vi "main--material example.vi"() -> ()   [LabVIEW 2021]
doc: "Example UI VI -- shows a couple example buttons and how to use the load and application VIs to theme the sample UI\n\n<b>Code Developed By:</b>\nTechnology Service Corporation\nwww.tsc.com/atcs\n\nDeveloper:\nDaniel Coons"
uses:
  src/Material Theme/Material Theme.lvclass
  user32.dll
panel:
  in  "tab control--Inverse Primary":enum32{"Page 1", "Page 2"}(tab)
  in  "File Path (theme)":path
  in  "theme-switch":bool
  out "status":string
  in  "filled--text--rectangular":bool
  in  "tonal--icons--rounded":bool
  in  "outline--text--rectangular":bool
  in  "FAB Button":bool
  in  "Close":bool
  out "header":bool
  # "control UI role = Secondary"
  # "Note:  run the VI to see dynamic theme in action!"
  # "Front Panel Rule: Surface"
  # "control UI role = Primary"
  # "control UI role = Primary"
  # "Decoration--Surface Container Low"
  # "control UI role = Tertiary"
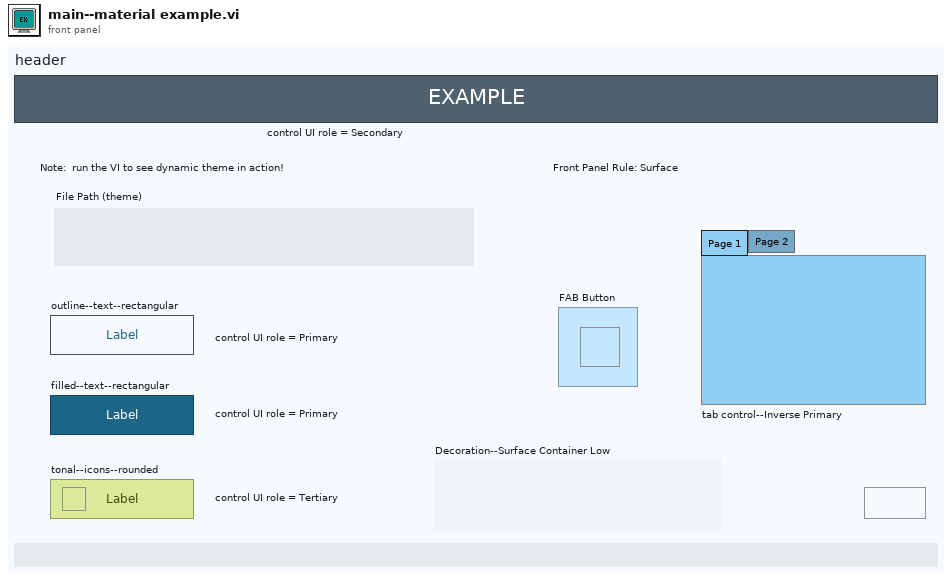
[diagram p1: front panel]
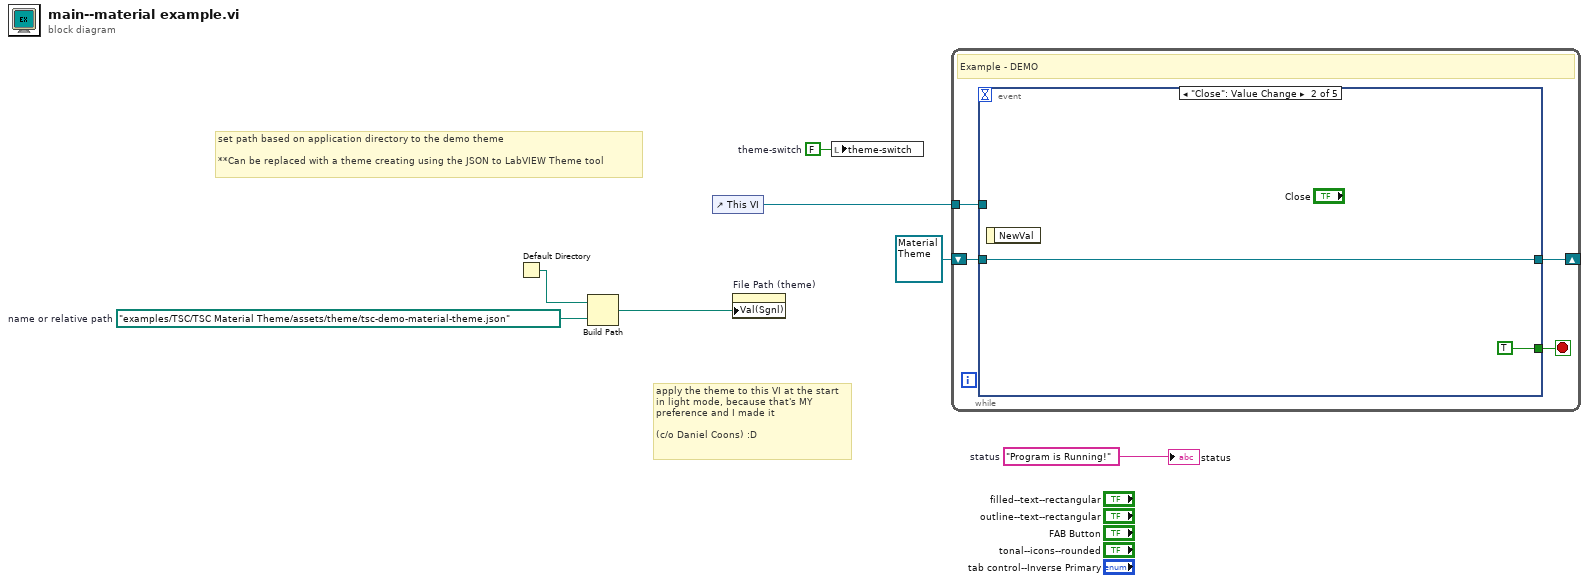
[diagram p0: block diagram]
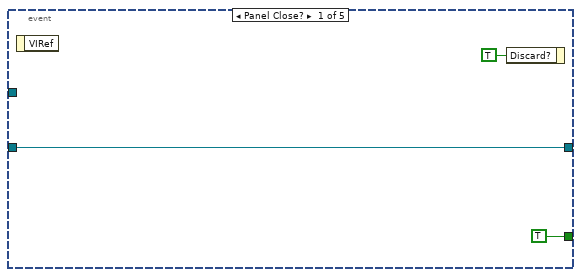
[diagram p2: hidden frame]
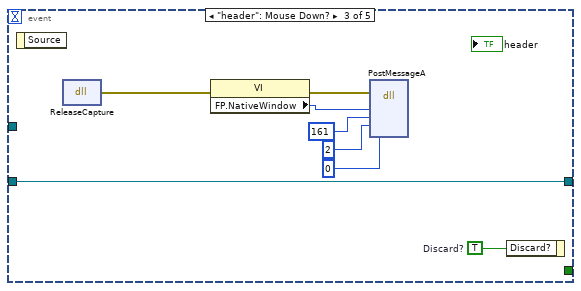
[diagram p3: hidden frame]
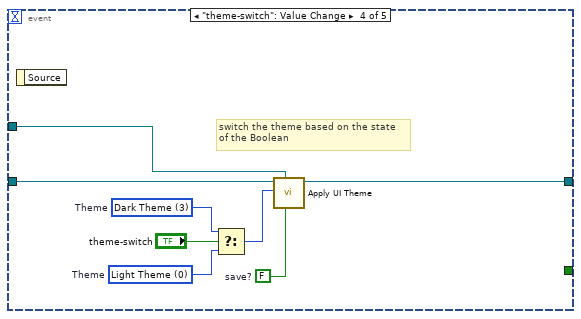
[diagram p4: hidden frame]
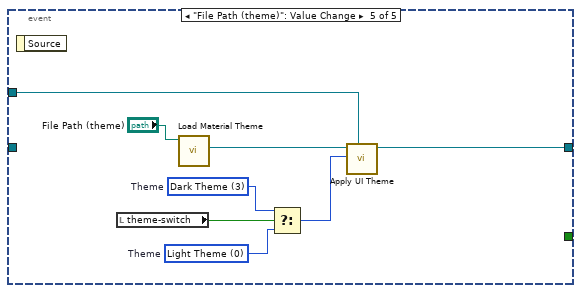
[diagram p5: hidden frame]
diagram:
  w4 = FALSE  # theme-switch
  w6 = path "examples/TSC/TSC Material Theme/assets/theme/tsc-demo-material-theme.json"  # name or relative path
  w7 = "Program is Running!"  # status
  # "apply the theme to this VI at the start\nin light mode, because that's MY \npreference and I made it\n\n(c/o Daniel Coons) :D"
  # "set path based on application directory to the demo theme\n\n**Can be replaced with a theme creating using the JSON to LabVIEW Theme tool"
  n1 = Default Directory() -> (w1:path)
  n2 = Build Path(base path=w1, name or relative path=w6) -> (appended path=w3:path)
  n3 = control-ref of="This VI"() -> (w5:refnum<vi>)
  n4 = property on="File Path (theme)" class="Path"("Val(Sgnl)"=w3) -> ()  [unwired: 2 in, 2 out]
  n5 = local write "theme-switch"(w4) -> ()
  n6 = while {
    tunnel: w5 -> [w9]
    shift-right: [w8] -> _
    shift-left: refnum<class "Material Theme.lvclass"> refnum ("Material Theme out") -> [w10]
    stop <- w11 stop-if-true
    # "Example - DEMO"
    n7 = event shown="[1] \"Close\": Value Change" {
      selector: _ -> [_ _ _ _ _]
      dyn-events: _ -> [_ _ _ _ _]
      timeout: _ -> [_ _ _ _ _]
      tunnel: [TRUE TRUE _ _ _] -> w11
      tunnel: w10 -> [w12 w15 w17 w32 _]
      tunnel: w9 -> [_ _ _ w31 w37]
      tunnel: [w12 w15 w17 w26 w38] -> w8
      event Panel Close? {
        n8 = event-data() -> ()  [unwired: 1 in, 1 out]
        n9 = event-data("Discard?"=TRUE) -> ()  [unwired: 1 in, 1 out]
      }
      event "Close": Value Change {
        n10 = event-data() -> ()  [unwired: 1 in, 1 out]
      }
      event "header": Mouse Down? {
        w24 = TRUE  # Discard?
        n11 = event-data() -> ()  [unwired: 1 in, 1 out]
        n12 = dll-call lib="user32.dll" fn="ReleaseCapture"() -> (error out=w20:errorcluster)  [unwired: 4 in, 1 out]
        n13 = property class="VI"(error in=w20) -> (error out=w19:errorcluster, "FP.NativeWindow"=w18:u64)  [unwired: 1 in, 1 out]
        n14 = dll-call lib="user32.dll" fn="PostMessageA"(error in=w19, "hWnd"=w18, "Msg"=161, "wParam"=2, "lParam"=0) -> ()  [unwired: 7 in, 2 out]
        n15 = event-data("Discard?"=w24) -> ()  [unwired: 1 in, 1 out]
      }
      event "theme-switch": Value Change {
        w25 = FALSE  # save?
        w29 = u16 3 items=["Light Theme", "Light Medium Contrast", "Light High Contrast", "Dark Theme", "Dark Medium Contrast", "Dark High Constrast"]  # Theme
        w28 = u16 0 items=["Light Theme", "Light Medium Contrast", "Light High Contrast", "Dark Theme", "Dark Medium Contrast", "Dark High Constrast"]  # Theme
        # "switch the theme based on the state\nof the Boolean"
        n16 = event-data() -> ()  [unwired: 1 in, 1 out]
        n17 = Select(t=w29, s="theme-switch", f=w28) -> (s? t:f=w27:u16)
        n18 = call "Apply UI Theme.vi"("save?"=w25, "VI Refnum"=w31, "Theme Mode"=w27, "Material Theme in"=w32) -> ("Material Theme out"=w26:refnum<class "Material Theme.lvclass">)  [unwired: 6 in, 1 out]
      }
      event "File Path (theme)": Value Change {
        w34 = u16 3 items=["Light Theme", "Light Medium Contrast", "Light High Contrast", "Dark Theme", "Dark Medium Contrast", "Dark High Constrast"]  # Theme
        w35 = u16 0 items=["Light Theme", "Light Medium Contrast", "Light High Contrast", "Dark Theme", "Dark Medium Contrast", "Dark High Constrast"]  # Theme
        n19 = event-data() -> ()  [unwired: 1 in, 1 out]
        n20 = local read "theme-switch"() -> (w36:bool)
        n21 = call "Load Material Theme.vi"("file path"="File Path (theme)") -> ("Theme"=w40:refnum<class "Material Theme.lvclass">)  [unwired: 8 in, 2 out]
        n22 = Select(t=w34, s=w36, f=w35) -> (s? t:f=w33:u16)
        n23 = call "Apply UI Theme.vi"("VI Refnum"=w37, "Theme Mode"=w33, "Material Theme in"=w40) -> ("Material Theme out"=w38:refnum<class "Material Theme.lvclass">)  [unwired: 7 in, 1 out]
      }
    }
  }
  "status" <- w7
